vi "FIP_ExcelWrite.vi"(6 "Case Selector T/F":bool, 7 "Flush Wait Time":i32, 9 "File Path":path, 10 "Data":sgl, 11 "Array In (Shift)":dbl[](array[numeric])) -> (3 "Array Out (Shift)":dbl[](array[numeric]))   [LabVIEW 2023]
uses:
  <vilib>/express/express signal manip/GetorSetDDTAttributes/Shared VIs/TimeType.ctl
  <vilib>/express/express signal manip/GetorSetDDTAttributes/Shared VIs/TimeMode Enum to Boolean.vi
  <vilib>/express/express shared/transition.llb/Dynamic To Waveform Array.vi
  <vilib>/express/express signal manip/GetorSetDDTAttributes/Set DDT Attributes/SetT0.vi
  <vilib>/express/express shared/transition.llb/Waveform Array To Dynamic.vi
  <vilib>/express/express signal manip/GetorSetDDTAttributes/Set DDT Attributes/Set DDT Properties.xnode
  <vilib>/express/express signal manip/GetorSetDDTAttributes/Shared VIs/GetSetShared.lvlib
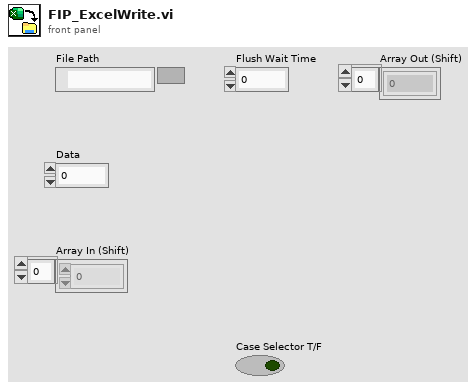
[diagram p1: front panel]
types:
  T1 = typedef "GetSetShared.lvlib/TimeType.ctl" = enum16{"Absolute", "Relative"}
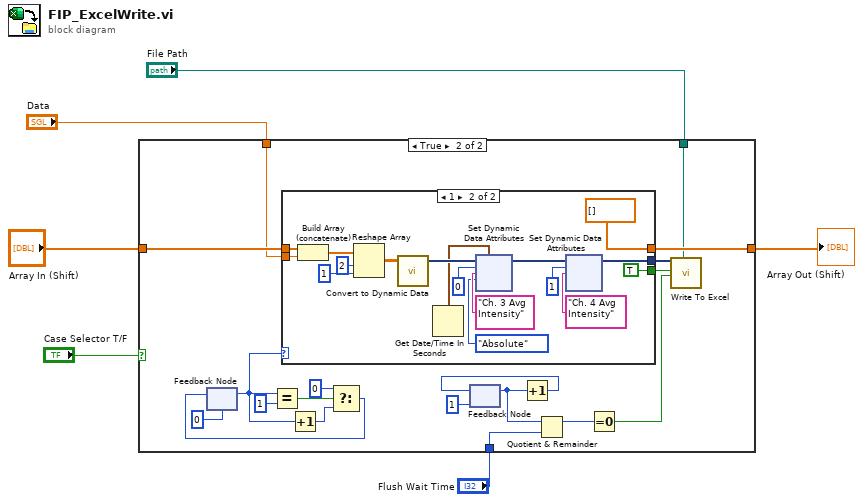
[diagram p0: block diagram]
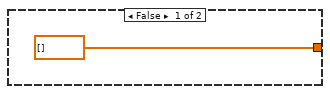
[diagram p2: hidden frame]
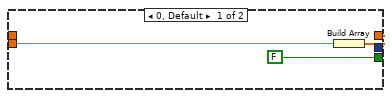
[diagram p3: hidden frame]
diagram:
  n1 = case shown="True" "Case Selector T/F" {
    tunnel: [dbl[] [] w22] -> w4
    tunnel: "Array In (Shift)" -> [_ w21]
    tunnel: "File Path" -> [_ w10]
    tunnel: "Data" -> [_ w9]
    tunnel: "Flush Wait Time" -> [_ w8]
    frame False {
    }
    frame True {
      n2 = feedback #1(0 ("dimension size")) -> (w14:i32)
      n3 = Equal?(x=w14, y=1) -> (x = y?=w19:bool)
      n4 = case shown="1" w14 {
        tunnel: w9 -> [w29 w45]
        tunnel: [w28 dbl[] []] -> w22
        tunnel: w21 -> [_ w46]
        tunnel: [FALSE ("Enable") TRUE ("Enable")] -> w24
        tunnel: [_ w32] -> w23
        frame 0, Default {
          n5 = Build Array(w29) -> (w28:sgl[])
        }
        frame 1 {
          n6 = Build Array (concatenate)(w46, w45) -> (w42:dbl[])
          n7 = Reshape Array(w42, 2 ("dimension size"), 1 ("dimension size")) -> (w39:dbl[][])
          n8 = call "Convert to Dynamic Data"("2D Array"=w39) -> ("Dynamic Data Type"=w38:dynamicdata)  [unwired: 3 in]
          n9 = Get Date/Time In Seconds() -> (seconds since 1Jan1904=w31:timestamp)
          n10 = xnode ("Set Dynamic Data Attributes")("Signals In"=w38, "Signal Index"=0, "Signal Name"="Ch. 3 Avg Intensity", "Time Mode"=TimeType."Absolute", "Timestamp"=w31) -> ("Signals Out"=w33:dynamicdata)  [unwired: 1 in, 1 out]
          n11 = xnode ("Set Dynamic Data Attributes")("Signals In"=w33, "Signal Index"=1, "Signal Name"="Ch. 4 Avg Intensity") -> ("Signals Out"=w32:dynamicdata)  [unwired: 3 in, 1 out]
        }
      }
      n12 = Increment(x=w14) -> (x+1=w15:i32)
      n13 = Select(t=0, s=w19, f=w15) -> (s? t:f=w16:i32)
      n14 = feedback-in #1(w16) -> ()
      n15 = feedback #2(1 ("dimension size")) -> (w12:i32)
      n16 = Increment(x=w12) -> (x+1=w11:i32)
      n17 = feedback-in #2(w11) -> ()
      n18 = Quotient & Remainder(x=w12, y=w8) -> (x-y*floor(x/y)=w26:i32)  [unwired: 1 out]
      n19 = Equal To 0?(x=w26) -> (x = 0?=w25:bool)
      n20 = call "Write To Excel"("Signals"=w23, "Enable"=w24, "Flush? (T)"=w25, "Filename"=w10) -> ()  [unwired: 13 in, 3 out]
    }
  }
  "Array Out (Shift)" <- w4
